vi "Tracking Test SAA.vi"(8 "error in (no error)":errorcluster, 10 "Model in":refnum<class "Model.lvclass">, 11 "Test Actuator State in":refnum<class "Test Actuator State.lvclass">) -> (0 "error out":errorcluster, 1 "Pass":bool, 2 "Model out":refnum<class "Model.lvclass">, 3 "Test Actuator State out":refnum<class "Test Actuator State.lvclass">)   [LabVIEW 2016, in "Test Actuator State.lvclass"]
uses:
  Test Actuator State.lvclass
  Model/Model/Model.lvclass
  <vilib>/Platform/TimedLoop/XDataNode/timing_clust.ctl
  <vilib>/Platform/TimedLoop/XDataNode/nitl_modes.ctl
  <vilib>/Platform/TimedLoop/XDataNode/wakeup.ctl
  Model/Model/Model.lvclass/Model.ctl
  Typedefs/ActuatorSetPoints.ctl
  <vilib>/Analysis/5stat.llb/RMS (DBL).vi
  <vilib>/Analysis/baseanly.llb/Mean (DBL).vi
  <vilib>/platform/TimedLoop/XDataNode/XDataNode.xnode
  Model/Waveforms/Waveform/Waveform.lvclass
  Typedefs/FAMT Typedefs.lvlib
  <vilib>/Analysis/NI_AALPro.lvlib
  <vilib>/Analysis/NI_AALBase.lvlib
  <vilib>/Platform/TimedLoop/XDataNode/XDNodeRunTimeDep.lvlib
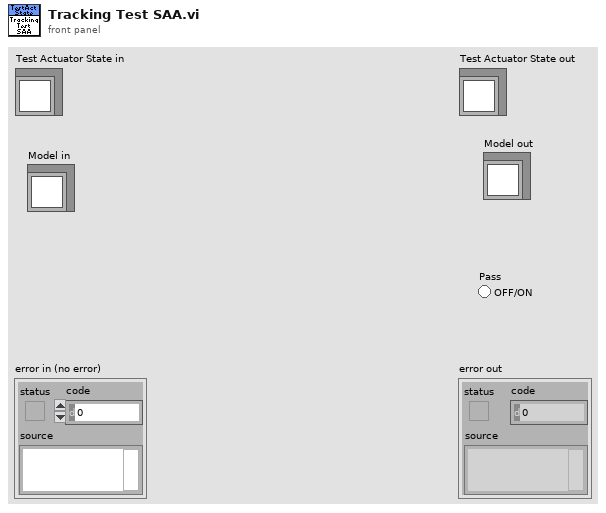
[diagram p1: front panel]
types:
  T1 = typedef "FAMT Typedefs.lvlib/TrackingTestSettings.ctl" = cluster{"Max Force Error (N)":dbl, "Max Moment (NM)":dbl, "Process Time (s)":dbl, "Sample Time (s)":dbl, "Iterations":i32, "Amplitude (N)":dbl, "Non-Repeating Error":dbl}
  T2 = typedef "XDNodeRunTimeDep.lvlib/timing_clust.ctl" = cluster{"Expected End [f-1]":u64, "Actual End [f-1]":u64, "Finished Late? [f-1]":bool, "Expected End [i-1]":u64, "Actual End [i-1]":u64, "Finished Late? [i-1]":bool, "Expected Start [i]":u64, "Actual Start [i]":u64, "Expected Start [f]":u64, "Actual Start [f]":u64, "Source Name":string, "Structure Name":string, "Period":i64, "Deadline":i64, "Offset":i64, "Start":i64, "Priority":i32, "Timeout":i32, "Mode":T3, "Wakeup Reason":T4, "Error":errorcluster, "Source Type":string, "Secondary Source Type":string, "Global End Time":u64, "Global Start Time":u64, "Frame Duration":u64, "Iteration Duration":u64, "Assigned CPU":i32, "I/O Scan Engine Mode":u32}
  T3 = typedef "XDNodeRunTimeDep.lvlib/nitl_modes.ctl" = enum32{"No Change", "Process missed periods, maintain original phase", "Discard missed periods, maintain original phase", "Process missed periods, ignore original phase", "Discard missed periods, ignore original phase"}
  T4 = typedef "XDNodeRunTimeDep.lvlib/wakeup.ctl" = enum32{"Normal", "Aborted", "Asynchronous wakeup", "Timing source error", "Timed loop error", "Timeout"}
  T5 = typedef "FAMT Typedefs.lvlib/ActuatorSetPoints.ctl" = cluster{"Axial Force":dbl, "Lateral Force":dbl, "FC1 Force":dbl, "FC2 Force":dbl}
  T6 = typedef "FAMT Typedefs.lvlib/ActuatorData.ctl" = cluster{"Timestamp":dbl, "Axial Force":dbl, "Lateral Force":dbl, "FC1 Force":dbl, "FC2 Force":dbl, "Lateral Push Pressure":dbl, "Lateral Pull Pressure":dbl, "Axial Push Pressure":dbl, "Axial Pull Pressure":dbl}
  T7 = typedef "FAMT Typedefs.lvlib/ToveyEngData.ctl" = cluster{"Timestamp":dbl, "Fx":dbl, "Fy":dbl, "Fz":dbl, "Mx":dbl, "My":dbl, "Mz":dbl}
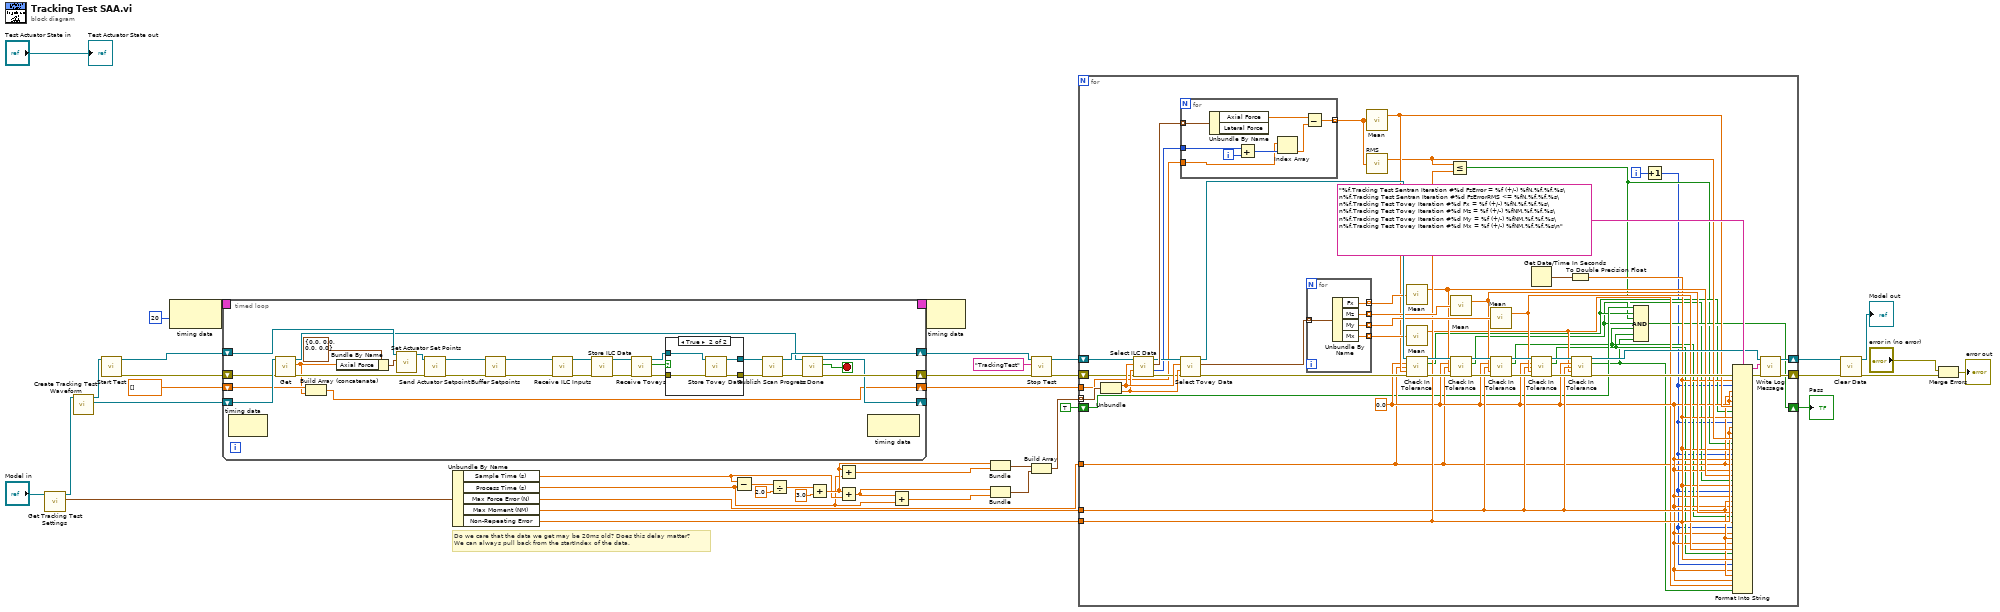
[diagram p0: block diagram]
diagram:
  # "Do we care that the data we get may be 20ms old? Does this delay matter?\nWe can always pull back from the startIndex of the data."
  n1 = call "Get Tracking Test Settings.vi"("Model in"="Model in") -> ("Tracking Test Settings"=w37:T1, "Model out"=w38:refnum<class "Model.lvclass">)  [unwired: 9 in]
  n2 = call "Create Tracking Test Waveform.vi"("Model in"=w38) -> ("Waveform"=w34:refnum<class "Waveform.lvclass">, "Model out"=w8:refnum<class "Model.lvclass">)  [unwired: 9 in]
  n3 = call "Start Test.vi"("Model in"=w8) -> ("error out"=w9:errorcluster, "Model out"=w10:refnum<class "Model.lvclass">)  [unwired: 9 in]
  n4 = node-c288(i64 20 ("Period")) -> (w13:T2)
  n5 = timed-loop {
    shift-right: [w69] -> w4
    shift-left: w10 -> [w61]
    shift-right: [w52] -> w2
    shift-left: w9 -> [w55]
    shift-right: [w50] -> _
    shift-left: w34 -> [w57]
    shift-right: [w47] -> w14
    shift-left: dbl[] [] -> [w49]
    timing: w13 -> [_]
    timing-out: [_] -> w12
    stop <- w51 stop-if-true
    n6 = node-c288() -> ()  [unwired: 1 in, 1 out]
    n7 = call-dynamic "Get.vi"("error in (no error)"=w55, "Waveform in"=w57) -> ("error out"=w54:errorcluster, "Value"=w48:dbl, "Waveform out"=w56:refnum<class "Waveform.lvclass">)  [unwired: 7 in]
    n8 = Build Array (concatenate)(w49, w48) -> (w47:dbl[])
    n9 = Bundle By Name(cluster=T5 {"Axial Force"=0.0, "Lateral Force"=0.0, "FC1 Force"=0.0, "FC2 Force"=0.0} ("Actuator Set Points"), "Axial Force"=w48) -> (w58:T5)
    n10 = call "Set Actuator Set Points.vi"("Actuator Set Points"=w58, "Model in"=w61) -> ("Model out"=w60:refnum<class "Model.lvclass">)  [unwired: 9 in]
    n11 = call "Send Actuator Setpoint.vi"("error in (no error)"=w54, "Model in"=w60) -> ("error out"=w43:errorcluster, "Model out"=w46:refnum<class "Model.lvclass">)  [unwired: 8 in]
    n12 = call "Buffer Setpoints.vi"("error in (no error)"=w43, "Model in"=w46) -> ("error out"=w44:errorcluster, "Model out"=w45:refnum<class "Model.lvclass">)  [unwired: 8 in]
    n13 = call "Receive ILC Inputs.vi"("error in (no error)"=w44, "Model in"=w45) -> ("error out"=w70:errorcluster, "Model out"=w71:refnum<class "Model.lvclass">)  [unwired: 8 in]
    n14 = call "Store ILC Data.vi"("error in (no error)"=w70, "Model in"=w71) -> ("error out"=w67:errorcluster, "Model out"=w68:refnum<class "Model.lvclass">)  [unwired: 8 in]
    n15 = call "Receive Toveys.vi"("error in (no error)"=w67, "Model in"=w68) -> ("error out"=w65:errorcluster, "Data Received"=w64:bool, "Model out"=w66:refnum<class "Model.lvclass">)  [unwired: 7 in]
    n16 = case shown="True" w64 {
      tunnel: w66 -> [w75 w79]
      tunnel: w65 -> [w74 w78]
      tunnel: [w74 w77] -> w62
      tunnel: [w75 w76] -> w63
      frame False {
      }
      frame True {
        n17 = call "Store Tovey Data.vi"("error in (no error)"=w78, "Model in"=w79) -> ("error out"=w77:errorcluster, "Model out"=w76:refnum<class "Model.lvclass">)  [unwired: 8 in]
      }
    }
    n18 = call "Publish Scan Progress.vi"("error in (no error)"=w62, "Model in"=w63) -> ("error out"=w53:errorcluster, "Model out"=w69:refnum<class "Model.lvclass">)  [unwired: 8 in]
    n19 = call-dynamic "Is Done.vi"("error in (no error)"=w53, "Waveform in"=w56) -> ("error out"=w52:errorcluster, "Is Done"=w51:bool, "Waveform out"=w50:refnum<class "Waveform.lvclass">)  [unwired: 7 in]
    n20 = node-c288() -> ()  [unwired: 1 in, 1 out]
  }
  n21 = Unbundle By Name(w37) -> ("Sample Time (s)"=w24:dbl, "Process Time (s)"=w22:dbl, "Max Force Error (N)"=w33:dbl, "Max Moment (NM)"=w16:dbl, "Non-Repeating Error"=w17:dbl)
  n22 = Subtract(x=w24, y=w22) -> (x-y=w30:dbl)
  n23 = Divide(x=w30, y=2.0) -> (x/y=w28:dbl)
  n24 = Add(x=w28, y=3.0) -> (x+y=w25:dbl)
  n25 = Add(x=w25, y=w22) -> (x+y=w26:dbl)
  n26 = Add(x=w25, y=w24) -> (x+y=w23:dbl)
  n27 = Add(x=w23, y=w22) -> (x+y=w21:dbl)
  n28 = node-c288(w12) -> ()  [unwired: 1 out]
  n29 = Bundle(w25, w26) -> (w20:cluster{dbl, dbl})  [unwired: 1 in]
  n30 = Bundle(w23, w21) -> (w19:cluster{dbl, dbl})  [unwired: 1 in]
  n31 = call "Stop Test.vi"("error in (no error)"=w2, "Test"="TrackingTest" ("format string"), "Model in"=w4) -> ("error out"=w1:errorcluster, "Model out"=w3:refnum<class "Model.lvclass">)  [unwired: 7 in]
  n32 = Build Array(w20, w19) -> (w18:cluster{dbl, dbl}[])
  n33 = for {
    tunnel: w18 -> [w134] mode=indexing
    shift-right: [w120] -> w31
    shift-left: w3 -> [w81]
    shift-right: [w121] -> w32
    shift-left: w1 -> [w80]
    tunnel: w33 -> [w91]
    tunnel: w16 -> [w96]
    tunnel: w17 -> [w101]
    tunnel: w14 -> [w93]
    shift-right: [w89] -> w6
    shift-left: TRUE -> [w90]
    i -> [w125]
    w95 = 0.0
    n34 = Unbundle(w134) -> (w131:dbl, w130:dbl)
    n35 = call "Select ILC Data.vi"("error in (no error)"=w80, "End Time"=w130, "Start Time"=w131, "Model in"=w81) -> ("error out"=w129:errorcluster, "StartIndex"=w92:i32, "Data"=w133:T6[], "Model out"=w132:refnum<class "Model.lvclass">)  [unwired: 4 in]
    n36 = for {
      tunnel: w133 -> [w147] mode=indexing
      tunnel: [w145] -> w104 mode=indexing
      tunnel: w93 -> [w141]
      tunnel: w92 -> [w144]
      i -> [w143]
      n37 = Unbundle By Name(w147) -> ("Axial Force"=w146:dbl)  [unwired: 1 out]
      n38 = Add(x=w144, y=w143) -> (x+y=w142:i32)
      n39 = Index Array(array=w141, index=w142) -> (element=w140:dbl)
      n40 = Subtract(x=w146, y=w140) -> (x-y=w145:dbl)
    }
    n41 = call "Select Tovey Data.vi"("error in (no error)"=w129, "End Time"=w130, "Start Time"=w131, "Model in"=w132) -> ("error out"=w123:errorcluster, "Data"=w128:T7[], "Model out"=w124:refnum<class "Model.lvclass">)  [unwired: 4 in, 1 out]
    n42 = for {
      tunnel: [w139] -> w116 mode=indexing
      tunnel: [w138] -> w115 mode=indexing
      tunnel: [w137] -> w112 mode=indexing
      tunnel: [w136] -> w109 mode=indexing
      tunnel: w128 -> [w135] mode=indexing
      n43 = Unbundle By Name(w135) -> ("Fx"=w139:dbl, "Mz"=w138:dbl, "My"=w137:dbl, "Mx"=w136:dbl)
    }
    n44 = call-poly <vilib>:"Mean.vi"("X"=w104) -> ("mean"=w103:dbl)  [unwired: 1 out]
    n45 = call-poly <vilib>:"RMS.vi"("X"=w104) -> ("rms value"=w102:dbl)  [unwired: 1 out]
    n46 = call-poly <vilib>:"Mean.vi"("X"=w116) -> ("mean"=w100:dbl)  [unwired: 1 out]
    n47 = call-poly <vilib>:"Mean.vi"("X"=w109) -> ("mean"=w94:dbl)  [unwired: 1 out]
    n48 = call "Check In Tolerance.vi"("Model in"=w124, "Expected"=w95, "Tolerance"=w91, "Actual"=w103, "error in (no error)"=w123) -> ("Model out"=w117:refnum<class "Model.lvclass">, "Pass"=w88:bool, "error out"=w118:errorcluster)  [unwired: 8 in]
    n49 = Less Or Equal?(x=w102, y=w101) -> (x <= y?=w87:bool)
    n50 = call-poly <vilib>:"Mean.vi"("X"=w115) -> ("mean"=w99:dbl)  [unwired: 1 out]
    n51 = call "Check In Tolerance.vi"("Model in"=w117, "Expected"=w95, "Tolerance"=w91, "Actual"=w100, "error in (no error)"=w118) -> ("Model out"=w114:refnum<class "Model.lvclass">, "Pass"=w86:bool, "error out"=w113:errorcluster)  [unwired: 8 in]
    n52 = call-poly <vilib>:"Mean.vi"("X"=w112) -> ("mean"=w98:dbl)  [unwired: 1 out]
    n53 = call "Check In Tolerance.vi"("Model in"=w114, "Expected"=w95, "Tolerance"=w96, "Actual"=w99, "error in (no error)"=w113) -> ("Model out"=w111:refnum<class "Model.lvclass">, "Pass"=w85:bool, "error out"=w110:errorcluster)  [unwired: 8 in]
    n54 = Get Date/Time In Seconds() -> (seconds since 1Jan1904=w126:timestamp)
    n55 = call "Check In Tolerance.vi"("Model in"=w111, "Expected"=w95, "Tolerance"=w96, "Actual"=w98, "error in (no error)"=w110) -> ("Model out"=w108:refnum<class "Model.lvclass">, "Pass"=w84:bool, "error out"=w106:errorcluster)  [unwired: 8 in]
    n56 = To Double Precision Float(number=w126) -> (double precision float=w97:dbl)
    n57 = call "Check In Tolerance.vi"("Model in"=w108, "Expected"=w95, "Tolerance"=w96, "Actual"=w94, "error in (no error)"=w106) -> ("Model out"=w107:refnum<class "Model.lvclass">, "Pass"=w83:bool, "error out"=w105:errorcluster)  [unwired: 8 in]
    n58 = Compound Arithmetic op=AND(w90, w88, w87, w86, w85, w84, w83) -> (w89:bool)
    n59 = Increment(x=w125) -> (x+1=w82:i32)
    n60 = Format Into String(format string="%f,Tracking Test Sentran Iteration #%d FzError = %f (+/-) %fN,%f,%f,%s\n%f,Tracking Test Sentran Iteration #%d FzErrorRMS <= %fN,%f,%f,%s\n%f,Tracking Test Tovey Iteration #%d Fx = %f (+/-) %fN,%f,%f,%s\n%f,Tracking Test Tovey Iteration #%d Mz = %f (+/-) %fNM,%f,%f,%s\n%f,Tracking Test Tovey Iteration #%d My = %f (+/-) %fNM,%f,%f,%s\n%f,Tracking Test Tovey Iteration #%d Mx = %f (+/-) %fNM,%f,%f,%s\n", error in=w105, w97, w82, w95, w91, w95, w103, w88, w97, w82, w101, w101, w102, w87, w97, w82, w95, w91, w95, w100, w86, w97, w82, w95, w96, w95, w99, w85, w97, w82, w95, w96, w95, w98, w84, w97, w82, w95, w96, w95, w94, w83) -> (resulting string=w119:string, error out=w122:errorcluster)  [unwired: 1 in]
    n61 = call "Write Log Message.vi"("error in (no error)"=w122, "Message"=w119, "Model in"=w107) -> ("error out"=w121:errorcluster, "Model out"=w120:refnum<class "Model.lvclass">)  [unwired: 7 in]
  }
  "Pass" <- w6
  n62 = call "Clear Data.vi"("error in (no error)"=w32, "Model in"=w31) -> ("error out"=w36:errorcluster, "Model out"=→"Model out":refnum<class "Model.lvclass">)  [unwired: 8 in]
  n63 = Merge Errors("error in (no error)", w36) -> (→"error out":errorcluster)
  "Test Actuator State out" <- "Test Actuator State in"
